vi "ShowRunningVIs.vi"() -> ()   [LabVIEW 2022 SP3, in "hse-misc.lvlib"]
doc: "Returns a list of VIs in memory\n\n\n\n____\nHAMPEL SOFTWARE ENGINEERING v3.8.0 (2023-12-18 14:41)"
uses:
  hse-misc.lvlib
panel:
  in  "Multicolumn Listbox":i32(listbox)
  in  "Stop?":bool
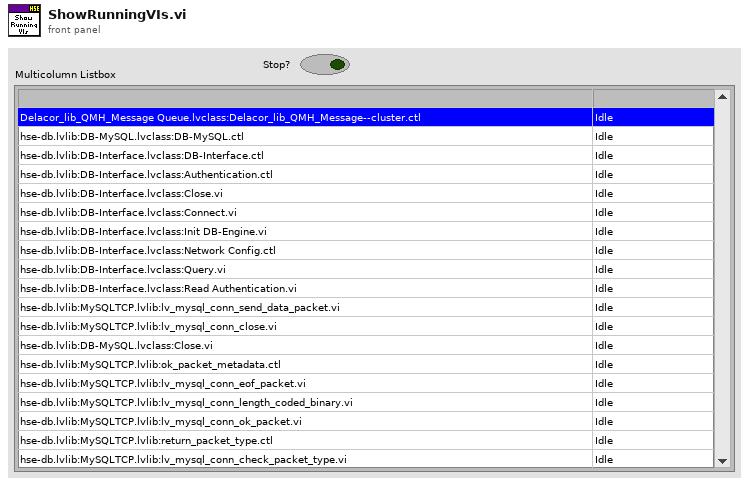
[diagram p1: front panel]
types:
  T1 = enum32{"Bad", "Idle", "Run top level", "Running"}
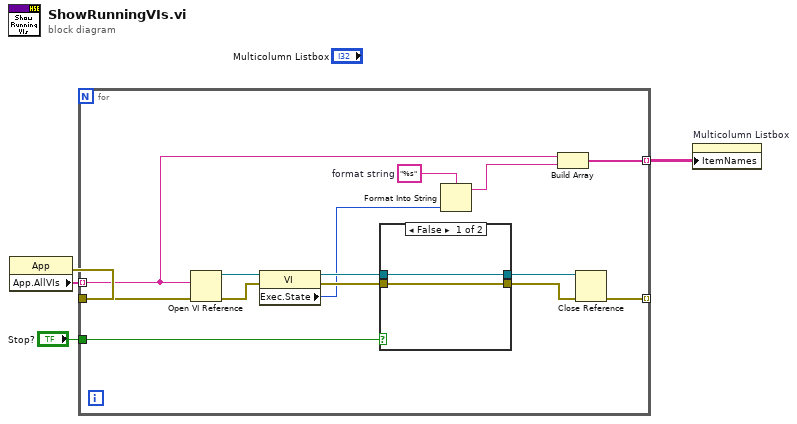
[diagram p0: block diagram]
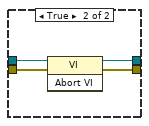
[diagram p2: hidden frame]
diagram:
  n1 = property class="App"() -> (error out=w3:errorcluster, "App.AllVIs"=w4:string[])  [unwired: 2 in, 1 out]
  n2 = for {
    tunnel: w4 -> [w9] mode=indexing
    tunnel: [w11] -> _ mode=indexing
    tunnel: w3 -> [w13]
    tunnel: "Stop?" -> [w12]
    tunnel: [w5] -> w1 mode=indexing
    w6 = "%s"  # format string
    n3 = Open VI Reference(vi path=w9, error in (no error)=w13) -> (vi reference=w18:refnum<vi>, error out=w16:errorcluster)  [unwired: 4 in]
    n4 = property class="VI"(reference=w18, error in=w16) -> (reference out=w17:refnum<vi>, error out=w15:errorcluster, "Exec.State"=w8:T1)
    n5 = case shown="False" w12 {
      tunnel: w17 -> [w19 w24]
      tunnel: w15 -> [w20 w23]
      tunnel: [w20 w22] -> w14
      tunnel: [w19 w21] -> w10
      frame False {
      }
      frame True {
        n6 = invoke class="VI" method="Abort VI"(reference=w24, error in=w23) -> (reference out=w21:refnum<vi>, error out=w22:errorcluster)  [unwired: 1 in, 1 out]
      }
    }
    n7 = Format Into String(format string=w6, w8) -> (resulting string=w7:string)  [unwired: 2 in, 1 out]
    n8 = Build Array(w9, w7) -> (w5:string[])
    n9 = Close Reference(reference=w10, error in (no error)=w14) -> (error out=w11:errorcluster)
  }
  n10 = property on="Multicolumn Listbox" class="MCListbox (strict)"("ItemNames"=w1) -> ()  [unwired: 2 in, 2 out]
